vi "Database_String_Converter_LV86.vi"(4 "String Input (date/timeyyyy-mm-dd hh:mm:ss)":string) -> (1 "String Output (mm/dd/yyyy hh:mm:ss AM/PM)":string)   [LabVIEW 2015]
doc: "This VI's purpose is to convert the 'date/timeyyyy-mm-dd hh:mm:ss' format string from the DB Tools Format Datetime Str.vi to the 'mm/dd/yyy hh:mm:ss AM/PM' format string to use as a SQL query.\n\nVI written by:\nErik Johnson\nApplications Engineer\nNational Instruments\n12/12/2006"
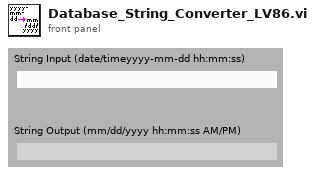
[diagram p1: front panel]
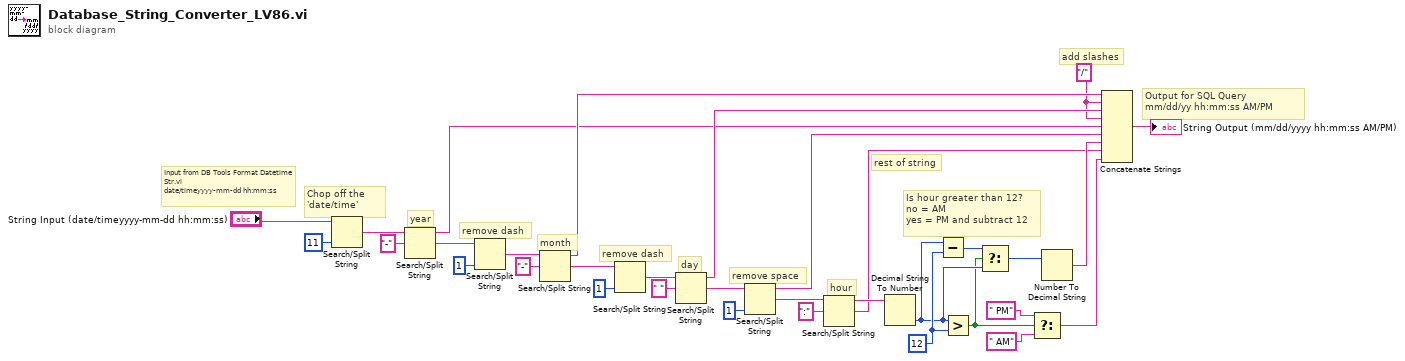
[diagram p0: block diagram]
diagram:
  w10 = 12 ("y")
  w18 = "/" ("string")
  # "Output for SQL Query\nmm/dd/yy hh:mm:ss AM/PM"
  # "Input from DB Tools Format Datetime Str.vi\ndate/timeyyyy-mm-dd hh:mm:ss"
  # "rest of string"
  # "Is hour greater than 12?\nno = AM\nyes = PM and subtract 12"
  # "hour"
  # "remove space"
  # "add slashes"
  # "day"
  # "month"
  # "remove dash"
  # "remove dash"
  # "year"
  # "Chop off the\n'date/time'"
  n1 = Search/Split String(string="String Input (date/timeyyyy-mm-dd hh:mm:ss)", offset (0)=11) -> (match + rest of string=w31:string)  [unwired: 3 out]
  n2 = Search/Split String(string=w31, search string/char (-)="-") -> (substring before match=w19:string, match + rest of string=w29:string)  [unwired: 2 out]
  n3 = Search/Split String(string=w29, offset (0)=1) -> (match + rest of string=w27:string)  [unwired: 3 out]
  n4 = Search/Split String(string=w27, search string/char (-)="-") -> (substring before match=w21:string, match + rest of string=w24:string)  [unwired: 2 out]
  n5 = Search/Split String(string=w24, offset (0)=1) -> (match + rest of string=w22:string)  [unwired: 3 out]
  n6 = Search/Split String(string=w22, search string/char (-)=" ") -> (substring before match=w20:string, match + rest of string=w16:string)  [unwired: 2 out]
  n7 = Search/Split String(string=w16, offset (0)=1) -> (substring before match=w11:string, match + rest of string=w15:string)  [unwired: 2 out]
  n8 = Search/Split String(string=w15, search string/char (-)=":") -> (substring before match=w13:string, match + rest of string=w3:string)  [unwired: 2 out]
  n9 = Decimal String To Number(string=w13) -> (number=w8:i32)  [unwired: 3 out]
  n10 = Subtract(x=w8, y=w10) -> (x-y=w7:i32)
  n11 = Greater?(x=w8, y=w10) -> (0:w6:bool)
  n12 = Select(t=w7, s=w6, f=w8) -> (s? t:f=w5:i32)
  n13 = Select(t=" PM" ("search string/char (-)"), s=w6, f=" AM" ("search string/char (-)")) -> (s? t:f=w2:string)
  n14 = Number To Decimal String(number=w5) -> (decimal integer string=w4:string)  [unwired: 1 out]
  n15 = Concatenate Strings(w21, w18, w20, w18, w19, w11, w4, w3, w2) -> (→"String Output (mm/dd/yyyy hh:mm:ss AM/PM)":string)
